vi "Separate Array Values.vi"(0 "输入数组":dbl[](array[numeric])=[6.0, 3.9, -5.8, 0.0, -2.6, -1.0, 2.2, -4.3] format="%0.2f") -> (1 "正数数组":dbl[](array[numeric]) format="%0.2f", 2 "负数数组":dbl[](array[numeric]) format="%0.2f")   [LabVIEW 2012]
doc: "该VI可将包含正数和负数的数组分解为分别包含正数和负数的两个数组。\n\nVI中包含“初始化数组”和“创建数组”函数，通过For循环自动索引输入数组。"
panel:
  # "本VI可将输入数组拆分为两个分别包含正数和负数的一维数组。"
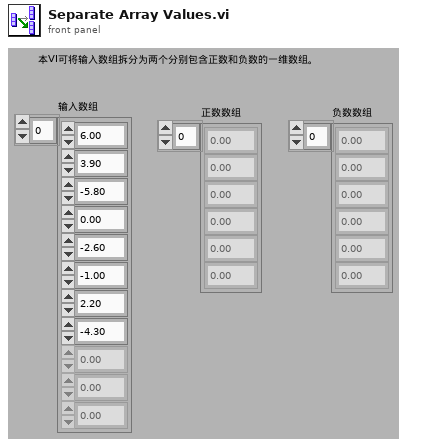
[diagram p1: front panel]
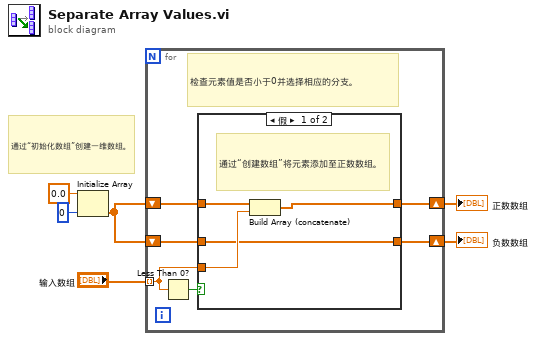
[diagram p0: block diagram]
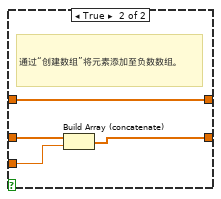
[diagram p2: hidden frame]
diagram:
  # "通过“初始化数组”创建一维数组。"
  n1 = Initialize Array(0.0, 0) -> (w6:dbl[])
  n2 = for {
    shift-right: [w10] -> w2
    shift-left: w6 -> [w9]
    shift-right: [w7] -> w1
    shift-left: w6 -> [w8]
    tunnel: "输入数组" -> [w11] mode=indexing
    # "检查元素值是否小于0并选择相应的分支。"
    n3 = Less Than 0? ("小于0？")(x=w11) -> (x < 0?=w12:bool)
    n4 = case shown="假" w12 {
      tunnel: w11 -> [w14 w19]
      tunnel: [w15 w20] -> w10
      tunnel: w9 -> [w16 w20]
      tunnel: w8 -> [w13 w18]
      tunnel: [w13 w17] -> w7
      frame False {
        # "通过“创建数组”将元素添加至正数数组。"
        n5 = Build Array (concatenate) ("创建数组")(w16, w14) -> (w15:dbl[])
      }
      frame True {
        # "通过“创建数组”将元素添加至负数数组。"
        n6 = Build Array (concatenate) ("创建数组")(w18, w19) -> (w17:dbl[])
      }
    }
  }
  "正数数组" <- w2
  "负数数组" <- w1
